vi "Close.vi"(8 "error in (no error)":errorcluster, 11 "MultiReader in":refnum<class "MultiReader.lvclass">) -> (0 "error out":errorcluster, 3 "MultiReader out":refnum<class "MultiReader.lvclass">)   [LabVIEW 2013, in "MultiReader.lvclass"]
doc: "Closes all open references and reserved resources for the reader"
uses:
  MultiReader.lvclass
  BaseReader/BaseReader.lvclass
  MultiReader.lvclass/MultiReader.ctl
  Message/VariantMessage/VariantMessage.lvclass
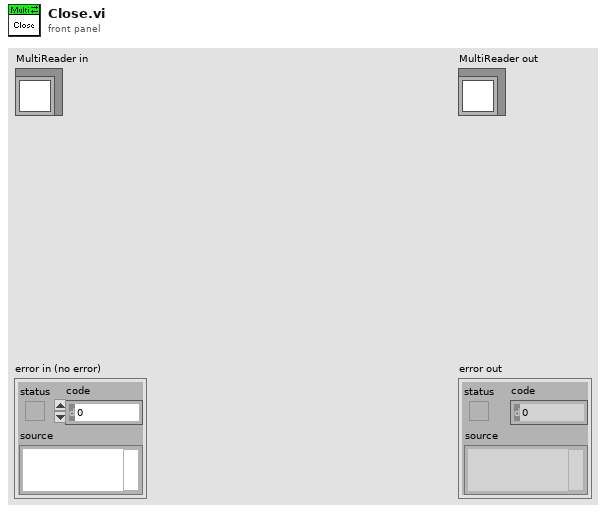
[diagram p1: front panel]
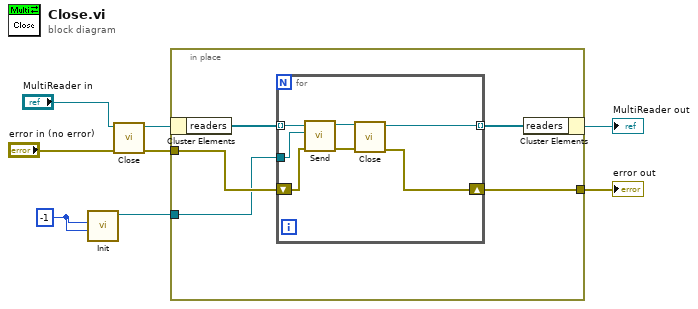
[diagram p0: block diagram]
diagram:
  w2 = -1 ("Type")
  n1 = call "Init.vi"("Data"=w2, "Type"=w2) -> ("VariantMessage out"=w1:refnum<class "VariantMessage.lvclass">)  [unwired: 8 in, 1 out]
  n2 = call-parent "Close.vi"("error in (no error)"="error in (no error)", "BaseReader in"="MultiReader in") -> ("error out"=w3:errorcluster, "BaseReader out"=w6:refnum<class "MultiReader.lvclass">)  [unwired: 8 in]
  n3 = in-place {
    in-place-border: [w11] -> w4
    in-place-border: w3 -> [w10]
    in-place-border: w1 -> [w9]
    n4 = in-place-cluster #1(w6) -> ("readers"=w13:refnum<class "BaseReader.lvclass">[])
    n5 = for {
      tunnel: w13 -> [w18] mode=indexing
      tunnel: [w20] -> w12 mode=indexing
      shift-right: [w19] -> w11
      shift-left: w10 -> [w16]
      tunnel: w9 -> [w14]
      n6 = call-dynamic "Send.vi"("error in (no error)"=w16, "Message"=w14, "BaseReader in"=w18) -> ("error out"=w15:errorcluster, "BaseReader out"=w17:refnum<class "BaseReader.lvclass">)  [unwired: 6 in, 1 out]
      n7 = call-dynamic "Close.vi"("error in (no error)"=w15, "BaseReader in"=w17) -> ("error out"=w19:errorcluster, "BaseReader out"=w20:refnum<class "BaseReader.lvclass">)  [unwired: 8 in]
    }
    n8 = in-place-cluster #1("readers"=w12) -> (→"MultiReader out":refnum<class "MultiReader.lvclass">)
  }
  "error out" <- w4
